vi "E_digitial_line_out.vi"(3 "error in":errorcluster, 4 "task/channels in":refnum<k21>, 5 "milliseconds to wait":u32, 6 "Boolean":bool) -> (0 "error out":errorcluster)   [LabVIEW 2013]
uses:
  <vilib>/DAQmx/write.llb/DAQmx Write (Digital Bool 1Line 1Point).vi
  <vilib>/DAQmx/miscellaneous.llb/DAQmx Fill In Error Info.vi
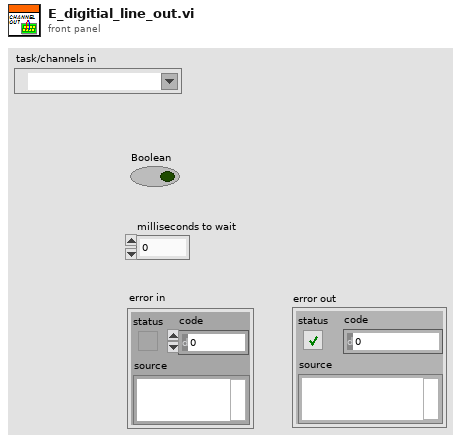
[diagram p1: front panel]
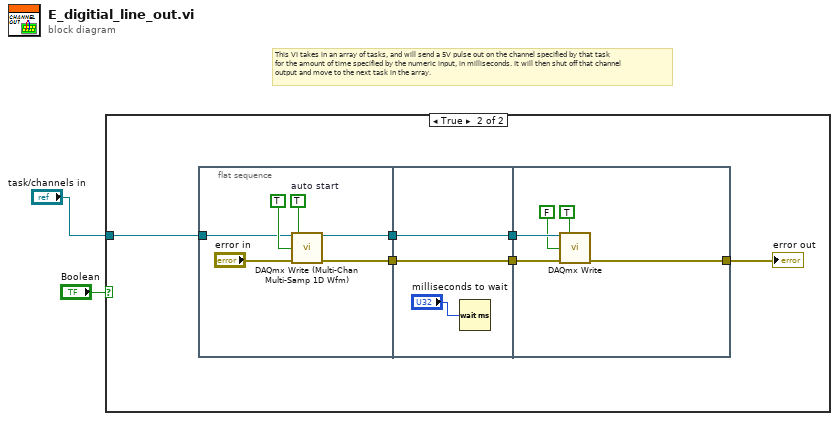
[diagram p0: block diagram]
diagram:
  # "This VI takes in an array of tasks, and will send a 5V pulse out on the channel specified by that task\nfor the amount of time specified by the numeric input, in milliseconds. It will then shut off that channel\noutput and move to the next task in the array."
  n1 = case shown="True" "Boolean" {
    tunnel: "task/channels in" -> [_ w3]
    frame False {
    }
    frame True {
      n2 = flat-sequence {
        tunnel: [w12] -> w7
        tunnel: [w11] -> w6
        tunnel: w3 -> [w9]
        tunnel: w7 -> [w17]
        tunnel: [w17] -> w5
        tunnel: [w15] -> w4
        tunnel: w6 -> [w15]
        tunnel: [w18] -> w8
        tunnel: w5 -> [w22]
        tunnel: w4 -> [w21]
        frame #0 {
          w14 = TRUE  # auto start
          n3 = call-poly "DAQmx Write (Multi-Chan Multi-Samp 1D Wfm).vi"("task/channels in"=w9, "auto start"=w14, "data"=TRUE, "error in"="error in") -> ("task out"=w11:refnum<k21>, "error out"=w12:errorcluster)  [unwired: 9 in, 1 out]
        }
        frame #1 {
          n4 = Wait (ms)(milliseconds to wait="milliseconds to wait") -> ()  [unwired: 1 out]
        }
        frame #2 {
          n5 = call-poly <vilib>:"DAQmx Write.vi"("task/channels in"=w21, "auto start"=TRUE, "data"=FALSE, "error in"=w22) -> ("error out"=w18:errorcluster)  [unwired: 9 in, 2 out]
        }
      }
      "error out" <- w8
    }
  }
